vi "MainV1.vi"() -> ()   [LabVIEW 2016]
uses:
  <vilib>/myRIO/Instrument Drivers/Onboard IO/AI/typedefs/AI Reference.ctl
  <vilib>/myRIO/Common/Instrument Driver Framework/Utilities/typedefs/myRIO Generic Hardware Reference.ctl
  <vilib>/myRIO/Common/Instrument Driver Framework/Utilities/typedefs/Hardware Version Enum.ctl
  <vilib>/myRIO/Common/Instrument Driver Framework/Utilities/typedefs/myRIO v1.0 Reference.ctl
  <vilib>/myRIO/Common/Instrument Driver Framework/Utilities/typedefs/Generic FPGA Reference.ctl
  <vilib>/myRIO/Common/Instrument Driver Framework/myRIO v1.0/AI/typedefs/AI Channels List.ctl
  <vilib>/myRIO/Common/Instrument Driver Framework/myRIO v1.0/AI/typedefs/AI Channels Enum.ctl
  <vilib>/myRIO/Common/Instrument Driver Framework/Utilities/typedefs/Analog Scaling Constants List.ctl
  <vilib>/myRIO/Common/Instrument Driver Framework/Utilities/typedefs/Analog Scaling Constants.ctl
  <vilib>/userdefined/High Color/nirio_resource_hc.ctl
  <vilib>/myRIO/Instrument Drivers/Onboard IO/PWM/typedefs/PWM Reference.ctl
  <vilib>/myRIO/Common/Instrument Driver Framework/myRIO v1.0/PWM/typedefs/PWM Channels Enum.ctl
  <vilib>/myRIO/Instrument Drivers/Onboard IO/PWM/typedefs/PWM Configuration.ctl
  <vilib>/myRIO/Common/Instrument Driver Framework/Utilities/vis/Is FPGA Ref Available.vi
  <vilib>/myRIO/Common/Instrument Driver Framework/myRIO v1.0/AI/vis/myRIO v1.1 Open AI.vi
  <vilib>/myRIO/Instrument Drivers/Onboard IO/AI/vis/Read.vi
  <vilib>/myRIO/Common/Instrument Driver Framework/myRIO v1.0/PWM/vis/myRIO v1.1 Open PWM.vi
  <vilib>/myRIO/Instrument Drivers/Onboard IO/PWM/vis/Set Duty Cycle and Frequency.vi
  <vilib>/myRIO/Common/Instrument Driver Framework/Utilities/vis/Validate Channels.vi
  <vilib>/myRIO/Common/Instrument Driver Framework/myRIO v1.0/AI/vis/myRIO v1.0 Reserve AI.vi
  <vilib>/myRIO/Common/Instrument Driver Framework/myRIO v1.0/PWM/vis/myRIO v1.0 Reserve PWM.vi
  <vilib>/myRIO/Common/Instrument Driver Framework/myRIO v1.0/AI/vis/myRIO v1.0 Build MUX Configuration AI.vi
  <vilib>/myRIO/Common/Instrument Driver Framework/myRIO v1.0/Resource Manager/vis/myRIO v1.0 Reserve Channel List.vi
  <vilib>/myRIO/Common/Instrument Driver Framework/myRIO v1.0/PWM/vis/myRIO v1.0 Build MUX Configuration PWM.vi
  <vilib>/myRIO/Common/Instrument Driver Framework/myRIO v1.0/Resource Manager/vis/myRIO v1.0 Reserve Channel.vi
  <vilib>/myRIO/Common/Instrument Driver Framework/myRIO v1.0/Resource Manager/vis/myRIO v1.0 Unreserve Channel.vi
  <vilib>/myRIO/Common/Instrument Driver Framework/myRIO v1.0/Resource Manager/vis/myRIO v1.0 Create Configuration List.vi
  <vilib>/myRIO/Common/Instrument Driver Framework/myRIO v1.0/Resource Manager/vis/myRIO v1.0 Build Mutex Name.vi
  <vilib>/Utility/VariantDataType/GetNumericInfo.vi
  <vilib>/Utility/error.llb/Error Cluster From Error Code.vi
  <vilib>/myRIO/Common/Instrument Driver Framework/myRIO v1.0/myRIO v1.1 Open.vi
  <vilib>/myRIO/Common/Instrument Driver Framework/Utilities/vis/IO Manager.vi
  <vilib>/myRIO/Common/Instrument Driver Framework/Utilities/vis/Configuration Manager.vi
  <vilib>/myRIO/Common/Instrument Driver Framework/myRIO v1.0/Resource Manager/vis/myRIO v1.0 Configure IO.vi
  <vilib>/myRIO/Common/Instrument Driver Framework/myRIO v1.0/myRIO v1.0 Close.vi
  <vilib>/myRIO/Common/Instrument Driver Framework/myRIO v1.0/PWM/vis/myRIO v1.0 Write PWM.vi
  <vilib>/myRIO/Common/Instrument Driver Framework/myRIO v1.0/AI/vis/myRIO v1.0 Get Scaling Constants AI.vi
  <vilib>/myRIO/Common/Instrument Driver Framework/myRIO v1.0/AI/vis/myRIO v1.0 Read AI.vi
  <vilib>/myRIO/Express VI/Onboard IO/PWM/PWM Express VI.xnode
  <vilib>/myRIO/Instrument Drivers/Onboard IO/PWM/vis/myRIO PWM Open.xnode
  <vilib>/myRIO/Express VI/Onboard IO/AI/AI Express VI.xnode
  <vilib>/myRIO/Instrument Drivers/Onboard IO/AI/vis/myRIO AI Open.xnode
  <vilib>/myRIO/Instrument Drivers/Onboard IO/PWM/PWM.lvlib
  <vilib>/myRIO/Instrument Drivers/Onboard IO/AI/AI.lvlib
panel:
  out "Rundenzeiten":T1={"Rundenzeiten[0]"=5.922, "Rundenzeiten[1]"=17.071, "Rundenzeiten[2]"=105.858, "Rundenzeiten[3]"=6.617, "Rundenzeiten[4]"=6.279, "Rundenzeiten[5]"=5.991, "Rundenzeiten[8]"=5.922}
  in  "PID Lenkung IR":T2={"proportional gain (Kc)"=0.5, "integral time (Ti, min)"=0.8, "derivative time (Td, min)"=0.002} {"derivative time (Td, min)" format="%.3f"; "integral time (Ti, min)" format="%.3f"; "proportional gain (Kc)" format="%.3f"}
  out "Impulse pro Minute":dbl
  out "counter":dbl=3364.0
  out "Leistung":dbl=-0.1536414641188581
  out "Linefollow_Array":bool[](array[boolean])
  in  "STOP if ON":bool
  in  "Geschwindigkeit multiplikator":dbl(knob) scale=0.0..1.0
  # "Minimum"
  # "immer nur 1 true!!!!!"
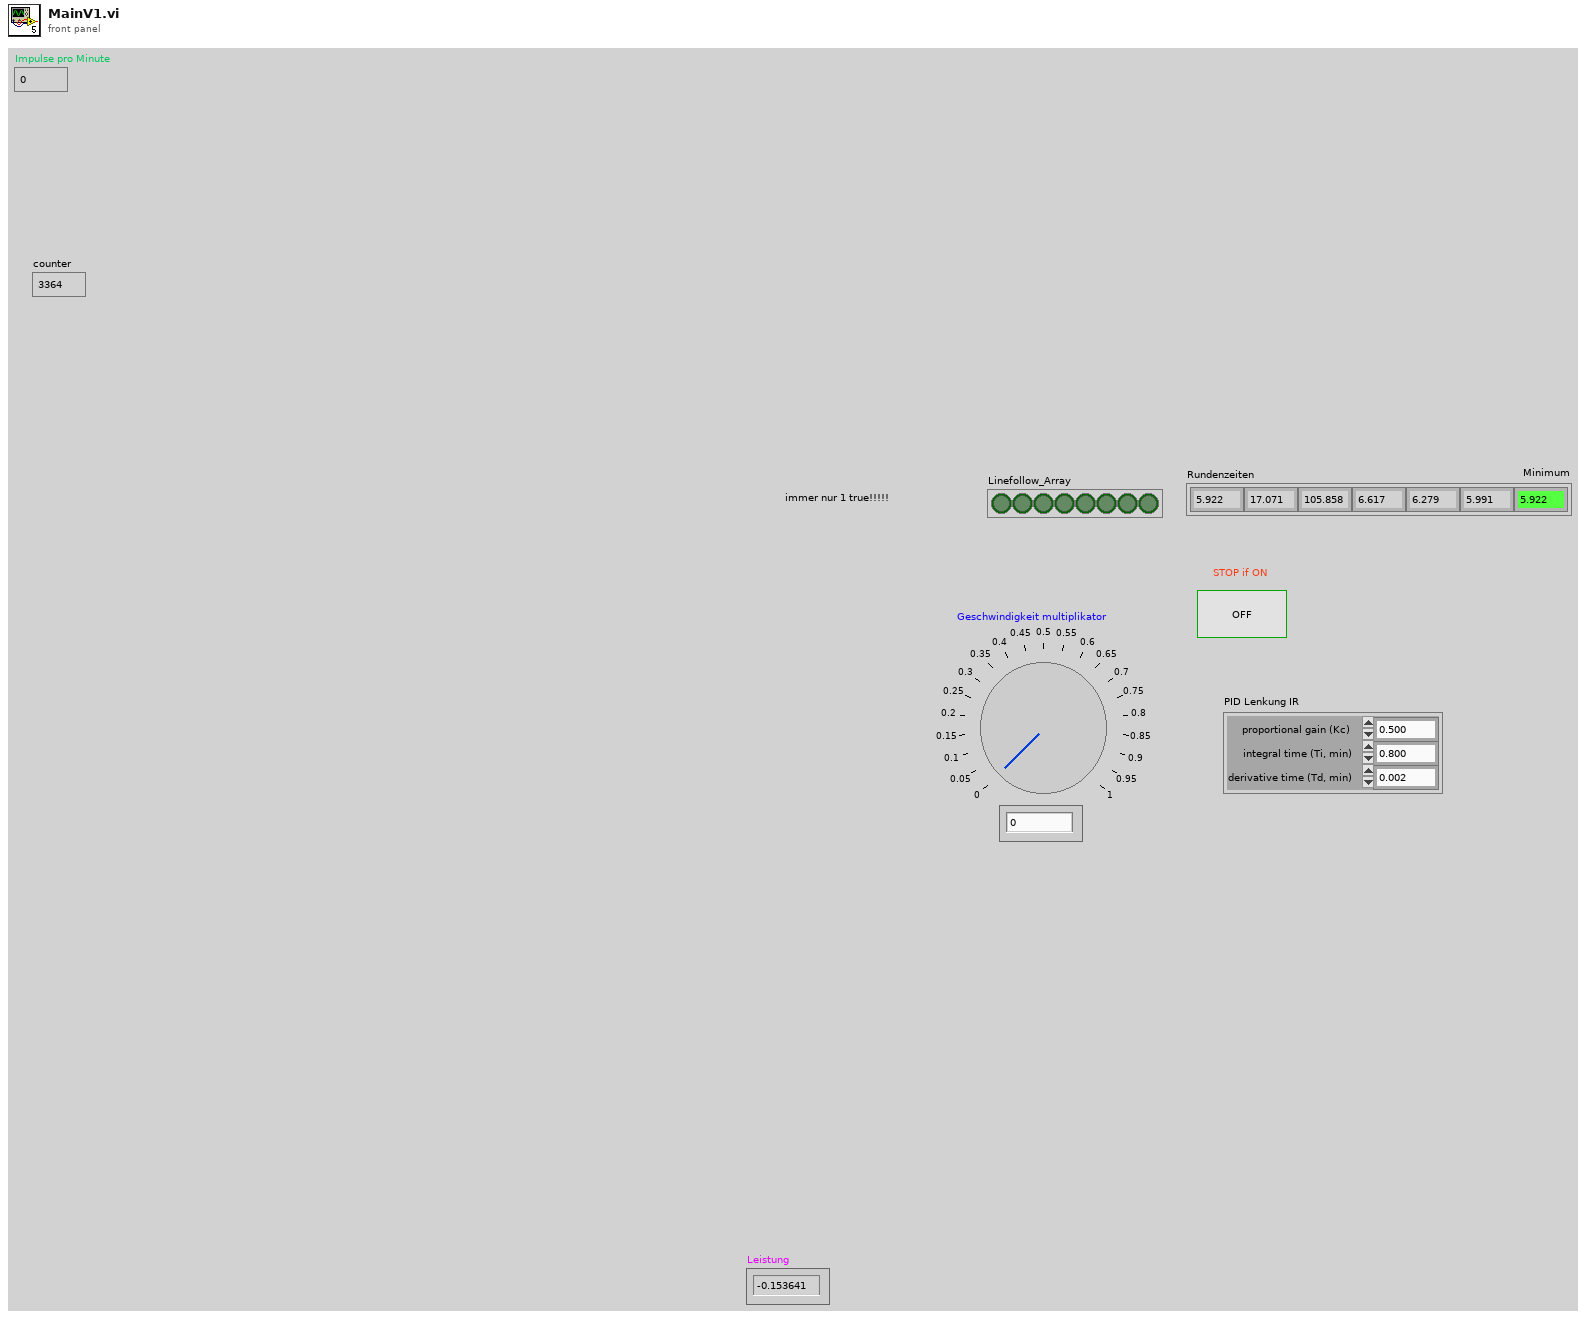
[diagram p1: front panel]
types:
  T1 = cluster{"Rundenzeiten[0]":dbl, "Rundenzeiten[1]":dbl, "Rundenzeiten[2]":dbl, "Rundenzeiten[3]":dbl, "Rundenzeiten[4]":dbl, "Rundenzeiten[5]":dbl, "Rundenzeiten[8]":dbl}
  T2 = cluster{"proportional gain (Kc)":dbl, "integral time (Ti, min)":dbl, "derivative time (Td, min)":dbl}
  T3 = typedef "PWM.lvlib/PWM Reference.ctl" = cluster{"myRIO Reference":T4, "PWM Channels Enum":T8, "PWM Configuration":T9}
  T4 = typedef "myRIO Generic Hardware Reference.ctl" = cluster{"myRIO Model":T5, "myRIO Hardware Reference":T6}
  T5 = typedef "Hardware Version Enum.ctl" = enum16{"Unknown", "myRIO-1900", "myRIO-1950", "roboRIO", "NI ELVIS RIO CM"}
  T6 = typedef "myRIO v1.0 Reference.ctl" = cluster{"Generic FPGA Reference":T7, "Allow multiple opens":bool}
  T7 = typedef "Generic FPGA Reference.ctl" = refnum<k20>
  T8 = typedef "PWM Channels Enum.ctl" = enum16{"Not Connected", "C/PWM0", "C/PWM1", "A/PWM0", "A/PWM1", "A/PWM2", "B/PWM0", "B/PWM1", "B/PWM2", "PWM/PWM0", "PWM/PWM1", "PWM/PWM2", "PWM/PWM3", "PWM/PWM4", "PWM/PWM5", "PWM/PWM6", "PWM/PWM7", "PWM/PWM8", "PWM/PWM9"}
  T9 = typedef "PWM.lvlib/PWM Configuration.ctl" = cluster{"Frequency":dbl, "Duty Cycle":dbl}
  T10 = typedef "nirio_resource_hc.ctl" = tag
  T11 = cluster{"Rundenzeiten[0]":dbl, "Rundenzeiten[1]":dbl, "Rundenzeiten[2]":dbl, "Rundenzeiten[3]":dbl, "Rundenzeiten[4]":dbl, "Rundenzeiten[5]":dbl, "Rundenzeiten[6]":dbl}
  T12 = typedef "AI.lvlib/AI Reference.ctl" = cluster{"myRIO Reference":T4, "AI Channels List":T13, "AI Scaling Constants List":T15}
  T13 = typedef "AI Channels List.ctl" = T14[]
  T14 = typedef "AI Channels Enum.ctl" = enum16{"Not Connected", "AudioIn/Left", "AudioIn/Right", "C/AI0", "C/AI1", "A/AI0", "A/AI1", "A/AI2", "A/AI3", "B/AI0", "B/AI1", "B/AI2", "B/AI3", "AI/AI0", "AI/AI1", "AI/AI2", "AI/AI3"}
  T15 = typedef "Analog Scaling Constants List.ctl" = T16[]
  T16 = typedef "Analog Scaling Constants.ctl" = cluster{"LSB Weight (Volts)":dbl, "Offset (Volts)":dbl, "Signed?":bool}
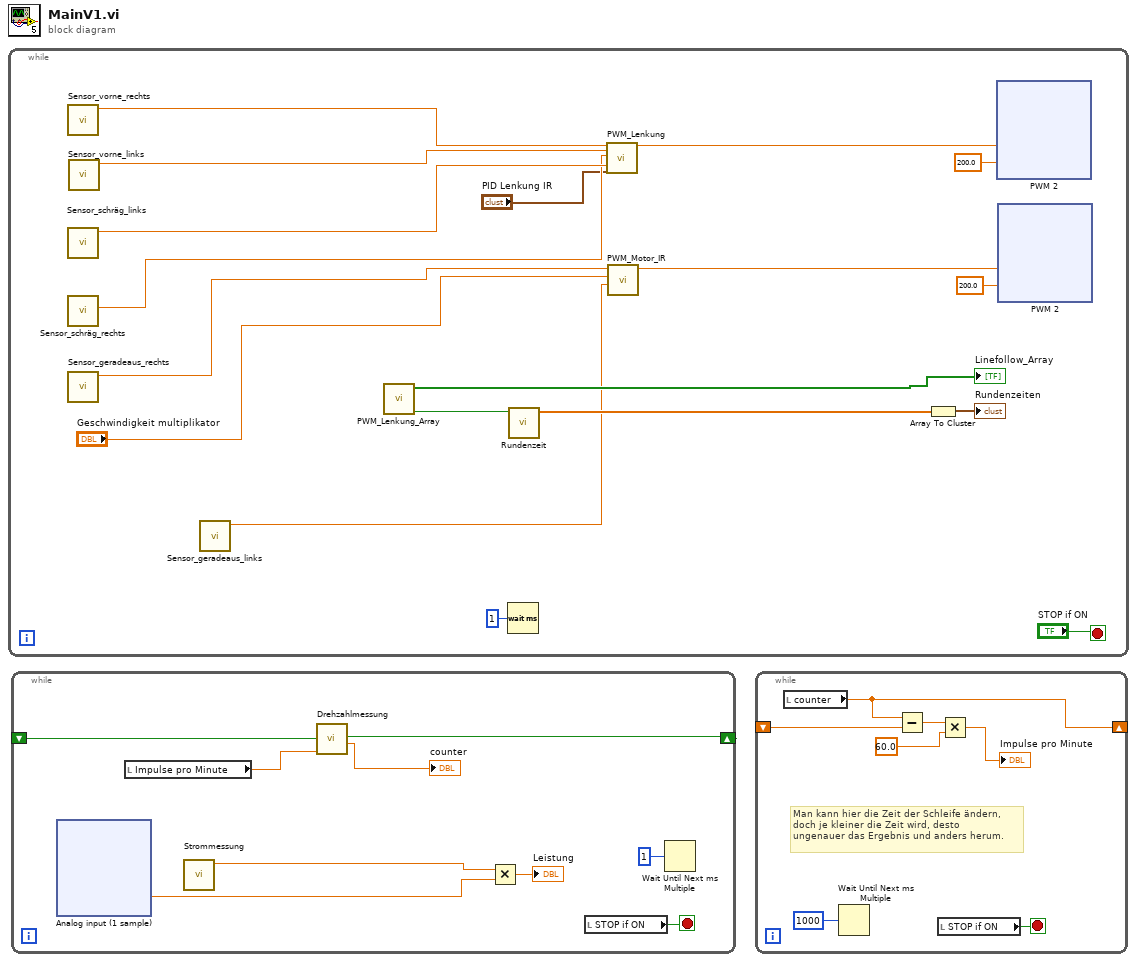
[diagram p0: block diagram]
diagram:
  n1 = while {
    stop <- "STOP if ON" stop-if-true
    n2 = call "Sensor_vorne_rechts.vi"() -> ("Abstand in cm"=w13:dbl)  [unwired: 11 in]
    n3 = call "Sensor_schräg_links.vi"() -> ("Abstand in cm"=w11:dbl)  [unwired: 11 in]
    n4 = call "Sensor_schräg_rechts.vi"() -> ("Abstand in cm"=w5:dbl)  [unwired: 11 in]
    n5 = call "Sensor_geradeaus_rechts.vi"() -> ("Abstand in cm"=w10:dbl)  [unwired: 11 in]
    n6 = call "Sensor_vorne_links.vi"() -> ("Abstand in cm"=w12:dbl)  [unwired: 11 in]
    n7 = call "Sensor_geradeaus_links.vi"() -> ("geradeaus links"=w1:dbl)  [unwired: 11 in]
    n8 = call "PWM_Lenkung_Array.vi"() -> ("8 IR true"=w2:bool, "Linefollow_Array"=→"Linefollow_Array":bool[])  [unwired: 8 in, 1 out]
    n9 = Wait (ms)(milliseconds to wait=u32 1) -> ()  [unwired: 1 out]
    n10 = call "Rundenzeit.vi"("8 IR true"=w2) -> ("Rundenzeiten"=w8:dbl[])  [unwired: 10 in]
    n11 = call "PWM_Lenkung.vi"("vorne rechts"=w13, "vorne links"=w12, "Schräg rechts"=w5, "Schräg links"=w11, "PID gains out 2"="PID Lenkung IR") -> ("PWM Lenkung"=w14:dbl)  [unwired: 14 in]
    n12 = call "PWM_Motor_IR.vi"("Sensorwert"=w10, "Geschwindigkeit multiplikator"="Geschwindigkeit multiplikator", "Sensorwert 2"=w1) -> ("PWM Motor"=w6:dbl)  [unwired: 6 in]
    n13 = Array To Cluster(array=w8) -> (cluster=→"Rundenzeiten":T11)
    n14 = xnode "PWM 2"("Duty Cycle"=w14, "Frequency [Hz]"=200.0 ("y")) -> ()  [unwired: 1 in, 1 out]
    n15 = xnode "PWM 2"("Duty Cycle"=w6, "Frequency [Hz]"=200.0) -> ()  [unwired: 1 in, 1 out]
  }
  n16 = while {
    shift-right: [w94] -> _
    shift-left: _ -> [w91]
    stop <- w89 stop-if-true
    n17 = xnode "Analog input (1 sample)"() -> ("C/AI0 (AI0)"=w93:dbl)  [unwired: 1 in, 1 out]
    n18 = local read "Impulse pro Minute"() -> (w96:dbl)
    n19 = call "Strommessung.vi"() -> ("Strom"=w90:dbl)  [unwired: 10 in, 1 out]
    n20 = call "Drehzahlmessung.vi"("Impuls per Minute"=w96, "in"=w91) -> ("counter"=→"counter":dbl, "out"=w94:bool)  [unwired: 6 in, 1 out]
    n21 = Multiply(x=w90, y=w93) -> (x*y=→"Leistung":dbl)
    n22 = local read "STOP if ON"() -> (w89:bool)
    n23 = Wait Until Next ms Multiple(millisecond multiple=u32 1 ("milliseconds to wait")) -> ()  [unwired: 1 out]
  }
  n24 = while {
    shift-right: [w140] -> _
    shift-left: _ -> [w139]
    stop <- w136 stop-if-true
    # "Man kann hier die Zeit der Schleife ändern, \ndoch je kleiner die Zeit wird, desto\nungenauer das Ergebnis und anders herum."
    n25 = local read "counter"() -> (w140:dbl)
    n26 = Wait Until Next ms Multiple(millisecond multiple=u32 1000 ("Vielfache von ms")) -> ()  [unwired: 1 out]
    n27 = Subtract(x=w140, y=w139) -> (x-y=w137:dbl)
    n28 = local read "STOP if ON"() -> (w136:bool)
    n29 = Multiply(x=w137, y=60.0) -> (x*y=→"Impulse pro Minute":dbl)
  }
